vi "Facade.vi"(0 "Data In":T7, 2 "Display State In":T2, 3 "Container State":T6) -> (6 "Data Out":T7, 7 "Display State Out":T2, 8 "Action":T1)   [LabVIEW 2020, in "SignalManager.xctl"]
uses:
  SignalManager.xctl
  Data.vi
  Classes/SignalManager/SignalManager.lvclass
  <vilib>/_xctls/Container State.ctl
  State.ctl
  Utility VIs/Controls/KListboxEx/Events.ctl
  Utility VIs/Controls/KListboxEx/Event Action.ctl
  PeriodDisplay.ctl
  Events.ctl
  Event Data.ctl
  <vilib>/_xctls/Action.ctl
  Utility VIs/Controls/KListboxEx/KListboxEx.xctl
  Channel/Channel.xctl
  Classes/Channel/Channel.lvclass
  Classes/Channel/Channel.lvclass/Channel.ctl
  Classes/SignalManager/SignalManager.lvclass/SignalManager.ctl
  Classes/Channel/Write Destination.vi
  Classes/SignalManager/Read Fs (Hz).vi
  Classes/SignalManager/Write Interval (ms).vi
  Classes/SignalManager/Read Interval (ms).vi
  Classes/SignalManager/Write Fs (Hz).vi
  Classes/SignalManager/Read Channels.vi
  Utility VIs/Math VIs/nearest multiple.vi
  <vilib>/_xctls/XControlSupport.lvlib
panel:
  in  "Sample rate (Hz)":dbl=1.0 format="%#_8g"
  in  "Channel":refnum<class "Channel.lvclass">(xcontrol)
  in  "Interval (ms)":dbl=1.0 format="%#_8g"
  in  "Rep rate (Hz)":dbl=1.0 format="%#.4g"
  in  "Channel List":i32(xcontrol)
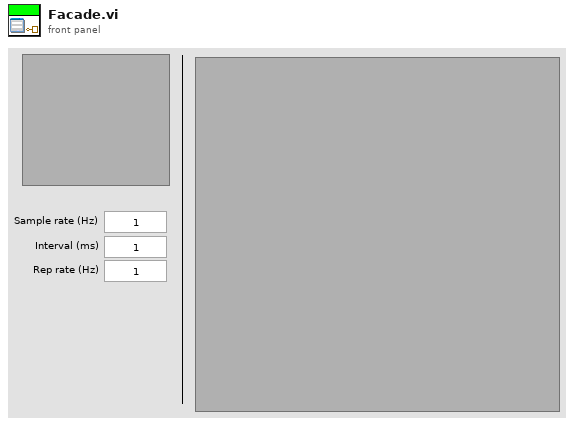
[diagram p1: front panel]
types:
  T1 = typedef "XControlSupport.lvlib/Action.ctl" = cluster{"Data Changed?":bool, "State Changed?":bool, "Action Name":string}
  T2 = typedef "SignalManager.xctl/State.ctl" = cluster{"Channels":T3, "Destinations":string[], "action":string, "EventReg":refnum<event-registration>, "selectedChan":i32, "Period Display":T4, "Events":T5, "Fs (Hz)":dbl, "TDT":bool, "Frame (ms)":dbl}
  T3 = typedef "KListboxEx.xctl/Events.ctl" = cluster{"Items Changed":refnum<user-event>, "List Changed":refnum<user-event>}
  T4 = typedef "SignalManager.xctl/PeriodDisplay.ctl" = enum16{"Interval", "RepRate", "Both", "Neither"}
  T5 = typedef "SignalManager.xctl/Events.ctl" = cluster{"Rename":refnum<user-event>}
  T6 = typedef "XControlSupport.lvlib/Container State.ctl" = cluster{"Indicator?":bool, "Run Mode?":bool, " Refnum":refnum<vi>}
  T7 = typedef "SignalManager.xctl/Data.vi" = refnum<class "SignalManager.lvclass">
  T8 = typedef "KListboxEx.xctl/Event Action.ctl" = enum16{"None", "Add", "Delete", "Move", "Edit", "Select"}
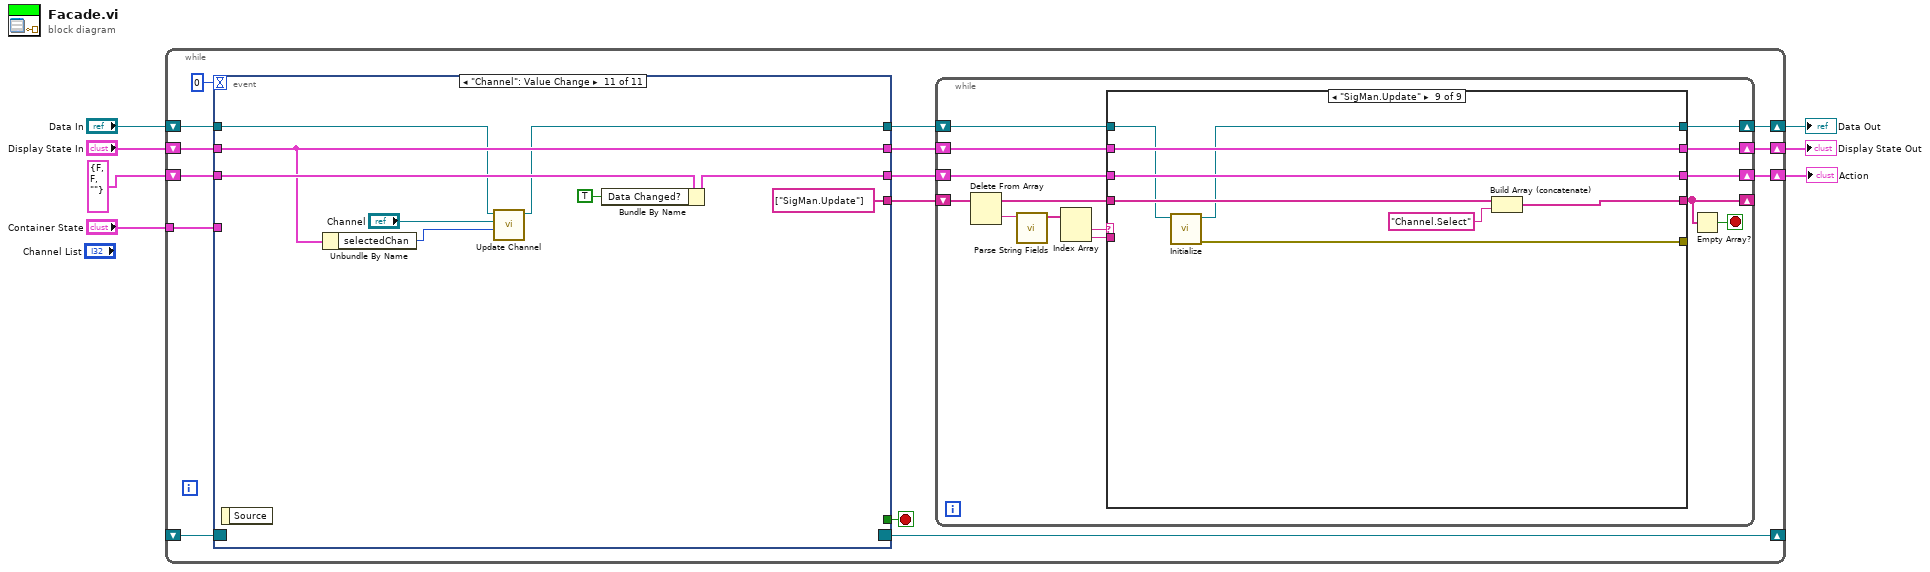
[diagram p0: block diagram]
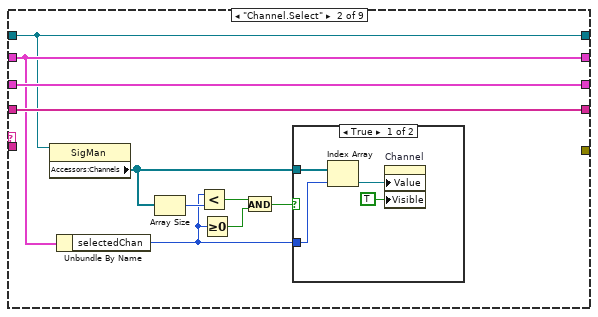
[diagram p3: hidden frame]
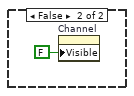
[diagram p4: hidden frame]
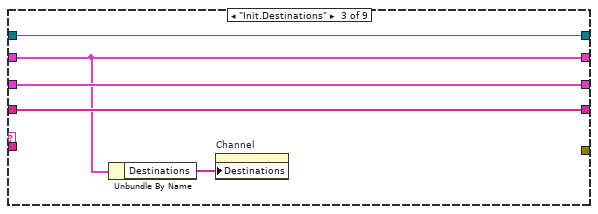
[diagram p5: hidden frame]
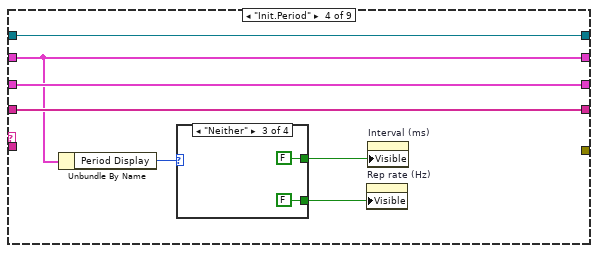
[diagram p6: hidden frame]
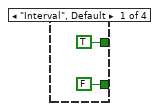
[diagram p7: hidden frame]
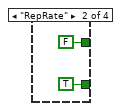
[diagram p8: hidden frame]
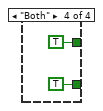
[diagram p9: hidden frame]
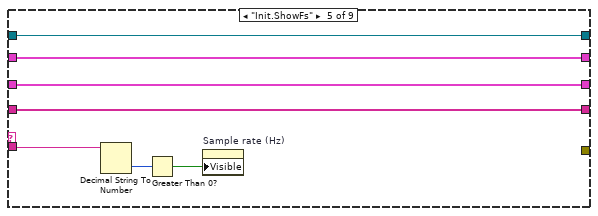
[diagram p10: hidden frame]
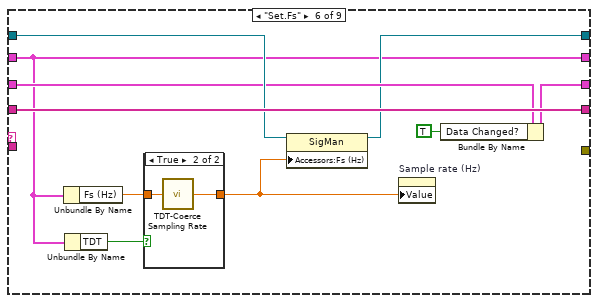
[diagram p11: hidden frame]
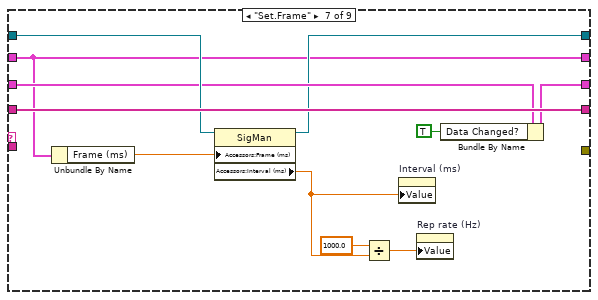
[diagram p13: hidden frame]
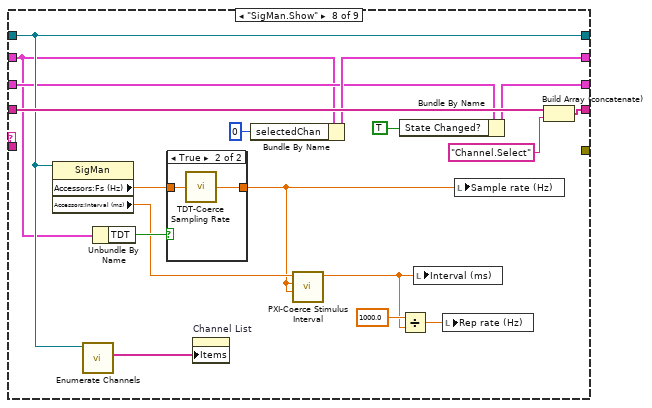
[diagram p14: hidden frame]
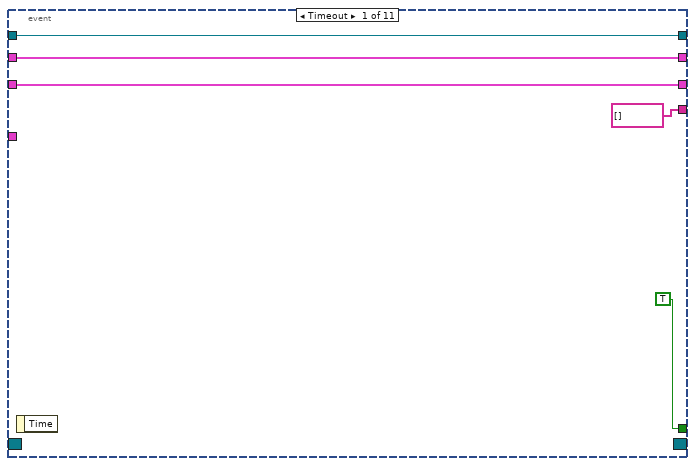
[diagram p16: hidden frame]
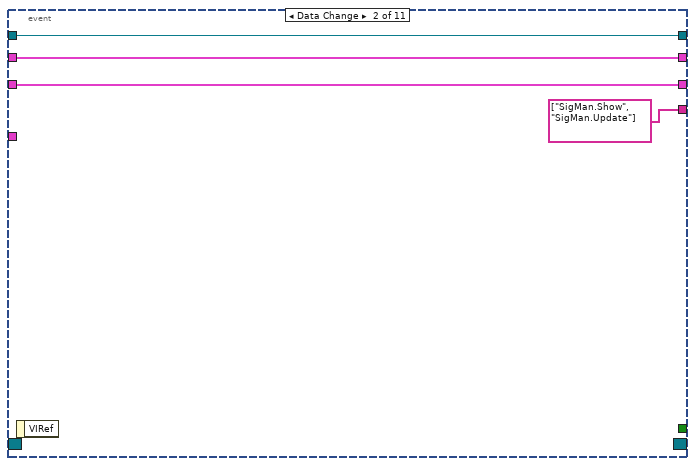
[diagram p17: hidden frame]
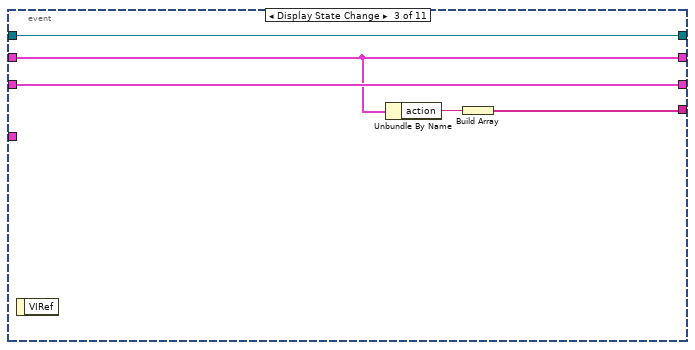
[diagram p18: hidden frame]
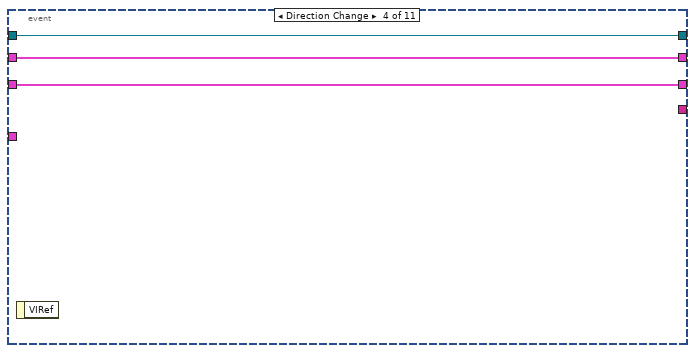
[diagram p19: hidden frame]
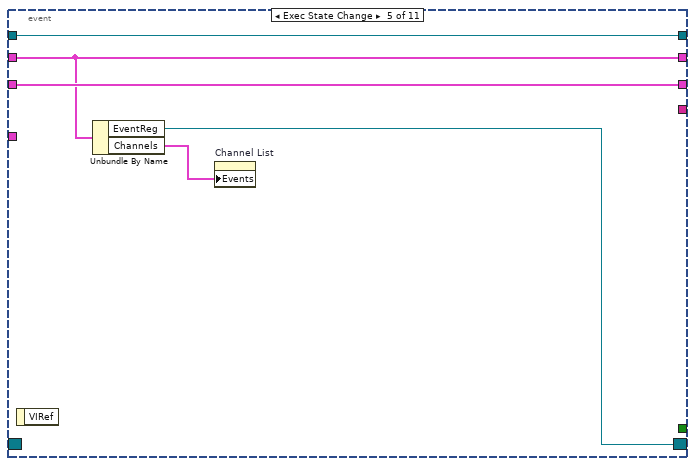
[diagram p20: hidden frame]
diagram:
  n1 = while {
    shift-right: [w11] -> w4
    shift-left: "Display State In" -> [w22]
    tunnel: "Container State" -> [w19]
    shift-right: [w12] -> w7
    shift-left: "Data In" -> [w18]
    shift-right: [w10] -> w2
    shift-left: T1 {"Data Changed?"=FALSE, "State Changed?"=FALSE, "Action Name"=""} ("Action") -> [w17]
    shift-right: [w9] -> _
    shift-left: _ -> [w8]
    stop <- w21 stop-if-true
    n2 = event shown="[10] \"Channel\": Value Change" {
      selector: w8 -> [_ _ _ _ _ _ _ _ _ _ _]
      dyn-events: [_ _ _ _ w153 _ _ _ _ _ _] -> w9
      timeout: 0 -> [_ _ _ _ _ _ _ _ _ _ _]
      tunnel: w22 -> [w138 w143 w147 w152 w155 w158 w207 w220 w223 w247 w255]
      tunnel: [w138 w143 w147 w152 w155 w158 w204 w220 w223 w247 w255] -> w14
      tunnel: [TRUE _ _ _ _ _ _ _ _ _ _] -> w21
      tunnel: w19 -> [_ _ _ _ _ _ _ _ _ _ _]
      tunnel: w18 -> [w137 w144 w149 w151 w157 w163 w206 w212 w229 w238 w252]
      tunnel: [w137 w144 w149 w151 w157 w162 w206 w218 w228 w245 w251] -> w15
      tunnel: [w139 w142 w148 w150 w156 w161 w202 w215 w227 w242 w250] -> w13
      tunnel: w17 -> [w139 w142 w148 w150 w156 w168 w205 w219 w230 w246 w256]
      tunnel: [string[] [] string[] ["SigMan.Show", "SigMan.Update"] w145 _ _ w159 string[] ["Channel.Select"] string[] ["SigMan.Update"] string[] ["SigMan.Update"] string[] ["SigMan.Update"] string[] ["SigMan.Update"]] -> w16
      event Timeout {
        n3 = event-data() -> ()  [unwired: 1 in, 1 out]
      }
      event Data Change {
        n4 = event-data() -> ()  [unwired: 1 in, 1 out]
      }
      event Display State Change {
        n5 = event-data() -> ()  [unwired: 1 in, 1 out]
        n6 = Unbundle By Name(w147) -> ("action"=w146:string)
        n7 = Build Array(w146) -> (w145:string[])
      }
      event Direction Change {
        n8 = event-data() -> ()  [unwired: 1 in, 1 out]
      }
      event Exec State Change {
        n9 = event-data() -> ()  [unwired: 1 in, 1 out]
        n10 = Unbundle By Name(w155) -> ("EventReg"=w153:refnum<event-registration>, "Channels"=w154:T3)
        n11 = property on="Channel List" class="KListboxEx (strict)"("Events"=w154) -> ()  [unwired: 2 in, 2 out]
      }
      event User Event {
        n12 = event-data() -> ("Action"=w167:T8, "Name"=w166:string, "Start row"=w165:i32, "End row"=w164:i32)  [unwired: 1 in]
        n13 = case shown="\"Add\"" w167 {
          tunnel: w166 -> [_ w180 w189 _]
          tunnel: w165 -> [_ w179 w193 w196]
          tunnel: w164 -> [_ _ _ _]
          tunnel: w163 -> [w169 w181 w195 w198]
          tunnel: [w169 w171 w194 w197] -> w162
          tunnel: [_ _ _ string[] ["Channel.Select"]] -> w159
          tunnel: w158 -> [_ w178 w192 _]
          frame "None", Default {
          }
          frame "Add" {
            n14 = Unbundle By Name(w178) -> ("Destinations"=w175:string[])
            n15 = call "Add Channel.vi"("Index"=w179, "Name"=w180, "SignalManager in"=w181) -> ("Channel"=w173:refnum<class "Channel.lvclass">, "SignalManager out"=w172:T7)  [unwired: 6 in, 1 out]
            n16 = Array Size(array=w175) -> (size(s)=w177:i32)
            n17 = Index Array(array=w175) -> (element=w174:string)  [unwired: 1 in]
            n18 = Equal?(x=w177, y=1) -> (x = y?=w170:bool)
            n19 = case shown="True" w170 {
              tunnel: w174 -> [_ w187]
              tunnel: w173 -> [_ w186]
              tunnel: w172 -> [w182 w185]
              tunnel: [w182 w183] -> w171
              frame False {
              }
              frame True {
                n20 = property class="Channel"(reference=w186, "Accessors:Destination"=w187) -> (reference out=w184:refnum<class "Channel.lvclass">)  [unwired: 1 in, 1 out]
                n21 = call "Update Channel (implicit).vi"("Channel"=w184, "SignalManager in"=w185) -> ("SignalManager out"=w183:T7)  [unwired: 8 in, 1 out]
              }
            }
          }
          frame "Edit" {
            n22 = Unbundle By Name(w192) -> ("Events.Rename"=w191:refnum<user-event>)
            n23 = call "Rename Channel.vi"("Index"=w193, "Name"=w189, "SignalManager in"=w195) -> ("Old name"=w190:string, "SignalManager out"=w194:T7)  [unwired: 6 in, 1 out]
            n24 = Bundle("Old name"=w190, "Name"=w189) -> (w188:cluster{"Old name":string, "Name":string})  [unwired: 1 in]
            n25 = Generate User Event(user event=w191, event data cluster=w188) -> ()  [unwired: 2 in, 2 out]
          }
          frame "Delete" {
            n26 = call "Delete Channel.vi"("Index"=w196, "SignalManager in"=w198) -> ("SignalManager out"=w197:T7)  [unwired: 8 in, 1 out]
          }
        }
        n27 = Bundle By Name(cluster=w168, "Data Changed?"=TRUE) -> (w161:T1)
      }
      event "Channel List": Value Change {
        n28 = event-data() -> ("NewVal"=w203:i32)  [unwired: 1 in]
        n29 = Bundle By Name(cluster=w207, "selectedChan"=w203) -> (w204:T2)
        n30 = Bundle By Name(cluster=w205, "State Changed?"=TRUE) -> (w202:T1)
      }
      event "Interval (ms)": Value Change {
        n31 = event-data() -> ()  [unwired: 1 in, 1 out]
        n32 = property class="SigMan"(reference=w212) -> ("Accessors:Fs (Hz)"=w211:dbl)  [unwired: 1 in, 2 out]
        n33 = call "PXI-Coerce Stimulus Interval.vi"("AI sampling rate (Hz)"=w211, "AO sampling rate (Hz)"=w211, "Stimulus interval (ms)"="Interval (ms)") -> ("Coerced interval (ms)"=w209:dbl)  [unwired: 5 in, 3 out]
        n34 = property class="SigMan"(reference=w212, "Accessors:Interval (ms)"=w209) -> (reference out=w218:T7, "Accessors:Interval (ms)"=w208:dbl)  [unwired: 1 in, 1 out]
        n35 = Divide(x=1000.0, y=w208) -> (x/y=w216:dbl)
        n36 = Bundle By Name(cluster=w219, "Data Changed?"=TRUE) -> (w215:T1)
        n37 = local write "Rep rate (Hz)"(w216) -> ()
        n38 = local write "Interval (ms)"(w208) -> ()
      }
      event "Sample rate (Hz)": Value Change {
        n39 = event-data() -> ()  [unwired: 1 in, 1 out]
        n40 = Unbundle By Name(w223) -> ("TDT"=w222:bool)
        n41 = case shown="True" w222 {
          tunnel: "Sample rate (Hz)" -> [w231 w233]
          tunnel: [w231 w232] -> w221
          frame False {
          }
          frame True {
            n42 = call "TDT-Coerce Sampling Rate.vi"("Fs (Hz)"=w233) -> ("Coerced"=w232:dbl)
          }
        }
        n43 = local write "Sample rate (Hz)"(w221) -> ()
        n44 = property class="SigMan"(reference=w229, "Accessors:Fs (Hz)"=w221) -> (reference out=w228:T7)  [unwired: 1 in, 1 out]
        n45 = Bundle By Name(cluster=w230, "Data Changed?"=TRUE) -> (w227:T1)
      }
      event "Rep rate (Hz)": Value Change {
        n46 = event-data() -> ()  [unwired: 1 in, 1 out]
        n47 = property class="SigMan"(reference=w238) -> ("Accessors:Fs (Hz)"=w239:dbl)  [unwired: 1 in, 2 out]
        n48 = Divide(x=1000.0, y="Rep rate (Hz)") -> (x/y=w237:dbl)
        n49 = call "PXI-Coerce Stimulus Interval.vi"("AI sampling rate (Hz)"=w239, "AO sampling rate (Hz)"=w239, "Stimulus interval (ms)"=w237) -> ("Coerced interval (ms)"=w235:dbl)  [unwired: 5 in, 3 out]
        n50 = property class="SigMan"(reference=w238, "Accessors:Interval (ms)"=w235) -> (reference out=w245:T7)  [unwired: 1 in, 1 out]
        n51 = local write "Interval (ms)"(w235) -> ()
        n52 = Divide(x=1000.0, y=w235) -> (x/y=w234:dbl)
        n53 = local write "Rep rate (Hz)"(w234) -> ()
        n54 = Bundle By Name(cluster=w246, "Data Changed?"=TRUE) -> (w242:T1)
      }
      event "Channel": Value Change {
        n55 = event-data() -> ()  [unwired: 1 in, 1 out]
        n56 = Unbundle By Name(w255) -> ("selectedChan"=w254:i32)
        n57 = call "Update Channel.vi"("Channel Index"=w254, "Channel"="Channel", "SignalManager in"=w252) -> ("SignalManager out"=w251:T7)  [unwired: 7 in, 1 out]
        n58 = Bundle By Name(cluster=w256, "Data Changed?"=TRUE) -> (w250:T1)
      }
    }
    n59 = while {
      shift-right: [w34] -> _
      shift-left: w16 -> [w36]
      shift-right: [w32] -> w12
      shift-left: w15 -> [w31]
      shift-right: [w30] -> w11
      shift-left: w14 -> [w29]
      shift-right: [w28] -> w10
      shift-left: w13 -> [w27]
      stop <- w33 stop-if-true
      n60 = Delete From Array(array=w36) -> (deleted portion=w25:string, array with subset deleted=w35:string[])  [unwired: 2 in]
      n61 = call "Parse String Fields.vi"("String"=w25) -> ("Fields"=w26:string[])  [unwired: 9 in, 1 out]
      n62 = Index Array(array=w26) -> (element #1=w24:string, element #2=w23:string)  [unwired: 2 in]
      n63 = case shown="\"SigMan.Update\"" w24 {
        tunnel: w35 -> [w40 w50 w60 w67 w82 w92 w106 w124 w135]
        tunnel: [w40 w50 w60 w67 w82 w92 w106 w120 w131] -> w34
        tunnel: [w37 w47 w59 w66 w81 w89 w103 w115 w128] -> w32
        tunnel: w31 -> [w37 w47 w59 w66 w81 w91 w105 w115 w132]
        tunnel: [w38 w48 w57 w64 w80 w86 w100 w121 w134] -> w30
        tunnel: w29 -> [w38 w48 w57 w64 w80 w86 w100 w111 w134]
        tunnel: [w39 w49 w58 w65 w79 w88 w102 w123 w133] -> w28
        tunnel: w27 -> [w39 w49 w58 w65 w79 w90 w104 w112 w133]
        tunnel: w23 -> [_ _ _ _ w77 _ _ _ _]
        tunnel: [_ _ _ _ _ _ _ _ w129] -> _
        frame "", Default {
        }
        frame "Channel.Select" {
          n64 = property class="SigMan"(reference=w47) -> ("Accessors:Channels"=w41:refnum<class "Channel.lvclass">[])  [unwired: 1 in, 2 out]
          n65 = Unbundle By Name(w48) -> ("selectedChan"=w43:i32)
          n66 = Array Size(array=w41) -> (size(s)=w46:i32)
          n67 = Less?(x=w43, y=w46) -> (x < y?=w45:bool)
          n68 = Greater Or Equal To 0?(x=w43) -> (x >= 0?=w44:bool)
          n69 = And(x=w45, y=w44) -> (x .and. y?=w42:bool)
          n70 = case shown="True" w42 {
            tunnel: w43 -> [w53 _]
            tunnel: w41 -> [w54 _]
            frame True {
              n71 = Index Array(array=w54, index=w53) -> (element=w52:refnum<class "Channel.lvclass">)
              n72 = property on="Channel" class="Channel (strict)"("Value"=w52, "Visible"=TRUE) -> ()  [unwired: 2 in, 2 out]
            }
            frame False {
              n73 = property on="Channel" class="Channel (strict)"("Visible"=FALSE) -> ()  [unwired: 2 in, 2 out]
            }
          }
        }
        frame "Init.Destinations" {
          n74 = Unbundle By Name(w57) -> ("Destinations"=w56:string[])
          n75 = property on="Channel" class="Channel (strict)"("Destinations"=w56) -> ()  [unwired: 2 in, 2 out]
        }
        frame "Init.Period" {
          n76 = Unbundle By Name(w64) -> ("Period Display"=w63:T4)
          n77 = case shown="\"Neither\"" w63 {
            tunnel: [TRUE FALSE FALSE TRUE] -> w62
            tunnel: [FALSE TRUE FALSE TRUE] -> w61
            frame "Interval", Default {
            }
            frame "RepRate" {
            }
            frame "Neither" {
            }
            frame "Both" {
            }
          }
          n78 = property on="Rep rate (Hz)" class="DigNum (strict)"("Visible"=w61) -> ()  [unwired: 2 in, 2 out]
          n79 = property on="Interval (ms)" class="DigNum (strict)"("Visible"=w62) -> ()  [unwired: 2 in, 2 out]
        }
        frame "Init.ShowFs" {
          n80 = Decimal String To Number(string=w77) -> (number=w78:i32)  [unwired: 2 in, 1 out]
          n81 = Greater Than 0?(x=w78) -> (x > 0?=w76:bool)
          n82 = property on="Sample rate (Hz)" class="DigNum (strict)"("Visible"=w76) -> ()  [unwired: 2 in, 2 out]
        }
        frame "Set.Fs" {
          n83 = Unbundle By Name(w86) -> ("Fs (Hz)"=w84:dbl)
          n84 = Unbundle By Name(w86) -> ("TDT"=w85:bool)
          n85 = case shown="True" w85 {
            tunnel: w84 -> [w93 w95]
            tunnel: [w93 w94] -> w83
            frame False {
            }
            frame True {
              n86 = call "TDT-Coerce Sampling Rate.vi"("Fs (Hz)"=w95) -> ("Coerced"=w94:dbl)
            }
          }
          n87 = property class="SigMan"(reference=w91, "Accessors:Fs (Hz)"=w83) -> (reference out=w89:T7)  [unwired: 1 in, 1 out]
          n88 = property on="Sample rate (Hz)" class="DigNum (strict)"("Value"=w83) -> ()  [unwired: 2 in, 2 out]
          n89 = Bundle By Name(cluster=w90, "Data Changed?"=TRUE) -> (w88:T1)
        }
        frame "Set.Frame" {
          n90 = Unbundle By Name(w100) -> ("Frame (ms)"=w99:dbl)
          n91 = property class="SigMan"(reference=w105, "Accessors:Frame (ms)"=w99) -> (reference out=w103:T7, "Accessors:Interval (ms)"=w98:dbl)  [unwired: 1 in, 1 out]
          n92 = Divide(x=1000.0, y=w98) -> (x/y=w97:dbl)
          n93 = property on="Interval (ms)" class="DigNum (strict)"("Value"=w98) -> ()  [unwired: 2 in, 2 out]
          n94 = property on="Rep rate (Hz)" class="DigNum (strict)"("Value"=w97) -> ()  [unwired: 2 in, 2 out]
          n95 = Bundle By Name(cluster=w104, "Data Changed?"=TRUE) -> (w102:T1)
        }
        frame "SigMan.Show" {
          n96 = property class="SigMan"(reference=w115) -> ("Accessors:Fs (Hz)"=w113:dbl, "Accessors:Interval (ms)"=w109:dbl)  [unwired: 1 in, 2 out]
          n97 = call "Enumerate Channels.vi"("SignalManager in"=w115) -> ("Names"=w114:string[])  [unwired: 8 in, 2 out]
          n98 = Unbundle By Name(w111) -> ("TDT"=w110:bool)
          n99 = case shown="True" w110 {
            tunnel: w113 -> [w125 w127]
            tunnel: [w125 w126] -> w108
            frame False {
            }
            frame True {
              n100 = call "TDT-Coerce Sampling Rate.vi"("Fs (Hz)"=w127) -> ("Coerced"=w126:dbl)
            }
          }
          n101 = property on="Channel List" class="KListboxEx (strict)"("Items"=w114) -> ()  [unwired: 2 in, 2 out]
          n102 = Bundle By Name(cluster=w111, "selectedChan"=0) -> (w121:T2)
          n103 = call "PXI-Coerce Stimulus Interval.vi"("AI sampling rate (Hz)"=w108, "AO sampling rate (Hz)"=w108, "Stimulus interval (ms)"=w109) -> ("Coerced interval (ms)"=w107:dbl)  [unwired: 5 in, 3 out]
          n104 = Bundle By Name(cluster=w112, "State Changed?"=TRUE) -> (w123:T1)
          n105 = Divide(x=1000.0, y=w107) -> (x/y=w116:dbl)
          n106 = local write "Interval (ms)"(w107) -> ()
          n107 = local write "Rep rate (Hz)"(w116) -> ()
          n108 = local write "Sample rate (Hz)"(w108) -> ()
          n109 = Build Array (concatenate)(w124, "Channel.Select") -> (w120:string[])
        }
        frame "SigMan.Update" {
          n110 = call "Initialize.vi"("SigMan in"=w132) -> ("error out"=w129:errorcluster, "SigMan out"=w128:T7)  [unwired: 9 in]
          n111 = Build Array (concatenate)(w135, "Channel.Select") -> (w131:string[])
        }
      }
      n112 = Empty Array?(array=w34) -> (empty?=w33:bool)
    }
  }
  "Display State Out" <- w4
  "Data Out" <- w7
  "Action" <- w2
